vi "Main.vi"(11 "Module Admin":refnum<class "Delacor_lib_QMH_Cloneable Module Admin.lvclass">) -> ()   [LabVIEW 2024, in "PLC.lvlib"]
doc: "This template is based off of the Queued Message Handler design pattern and the Queued Message Handler project template that ships with LabVIEW.\n\nThe main difference is that the queue is private to this module and communication between modules is performed via Broadcast and Request events.\n\nRequest events are wrapped in public API methods and are handled in the Event Handling Loop (EHL) of this VI. Any module can register for Broadcast events sent by this module. The EHL generates messages based on user interface actions.\n\nThe Message Handling Loop (MHL) processes messages generated by the EHL, or by other messages. The messages are string values, so new messages can be added easily to the Message Cases case structure in the MHL. Each message cluster can also provide an optional value for Message Data, which is a variant that can be converted to whatever message-specific data is required.\n_____\nBased on DQMH Dev Tools: Project Template 7.1.0.1503."
uses:
  PLC.lvlib
  <vilib>/Delacor/Delacor QMH/Libraries/Cloneable Module Admin_class/Delacor_lib_QMH_Cloneable Module Admin.lvclass
  C:/Program Files (x86)/National Instruments/LabVIEW 2024/vi.lib/Delacor/Delacor QMH/Libraries/Module Admin_class/Delacor_lib_QMH_Module Admin.lvclass
  Module Data--cluster.ctl
  <vilib>/Delacor/Delacor QMH/Libraries/Message Queue_class/Delacor_lib_QMH_Message Queue.lvclass/Delacor_lib_QMH_Message Queue.ctl
  <vilib>/Delacor/Delacor QMH/Libraries/Cloneable Module Admin_class/Delacor_lib_QMH_Cloneable Module Admin.lvclass/Delacor_lib_QMH_Cloneable Module Admin.ctl
  Stop Argument--cluster.ctl
  <vilib>/Delacor/Delacor QMH/Libraries/Module Admin_class/Delacor_lib_QMH_Module Admin.lvclass/Delacor_lib_QMH_Module Admin.ctl
  Set IP Argument--cluster.ctl
  Connect Argument--cluster.ctl
  Connect (Reply Payload)--cluster.ctl
  <vilib>/Utility/miscctls.llb/LVPointTypeDef.ctl
  <vilib>/Delacor/Delacor QMH/Libraries/Message Queue_class/Delacor_lib_QMH_Enqueue Message (Single).vi
  <vilib>/Delacor/Delacor QMH/Libraries/Cloneable Module Admin_class/Delacor_lib_QMH_Get Module ID.vi
  <vilib>/Delacor/Delacor QMH/Libraries/Module Admin_class/Delacor_lib_QMH_Get External Launch.vi
  <vilib>/NI/Modbus Library/API/Wrapper/Create TCP Master.vi
  <vilib>/Delacor/Delacor QMH/Libraries/Message Queue_class/Delacor_lib_QMH_Message Queue.lvclass
  <vilib>/NI/Modbus Library/API/Master/Modbus Master.lvclass
  <vilib>/NI/Modbus Library/API/Wrapper/API Main.lvlib
panel:
  out "discrete inputs":bool[](array[boolean])
  out "Timeout":bool
  out "Port":i32
  out "IP":string
  out "error out":errorcluster
  out "Status":string
  in  "Simulate EHL Error":bool
  in  "Simulate MHL Error":bool
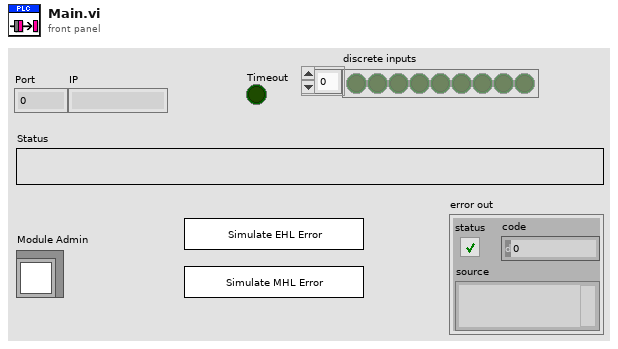
[diagram p1: front panel]
types:
  T1 = typedef "PLC.lvlib/Request Events--cluster.ctl" = cluster{"Stop Module":refnum<user-event>, "Show Panel":refnum<user-event>, "Hide Panel":refnum<user-event>, "Show Diagram":refnum<user-event>, "Get Module Execution Status":refnum<user-event>, "Set IP":refnum<user-event>, "Connect":refnum<user-event>, "Local Instance":T2}
  T2 = typedef "PLC.lvlib/Local Instance Request Events--cluster.ctl" = cluster{"Wake Up HL":refnum<user-event>}
  T3 = typedef "PLC.lvlib/Module Data--cluster.ctl" = cluster{"Status":string, "IP":string, "Port":i32}
  T4 = enum32{"invalid lock state", "Not Locked", "Locked (No Password)", "Password-protected"}
  T5 = typedef "PLC.lvlib/Stop Argument--cluster.ctl" = cluster{"Module ID":i32, "Origin":string, "Exit via Stop Module Req?":bool, "Wait for Module to stop?":bool}
  T6 = typedef "PLC.lvlib/Set IP Argument--cluster.ctl" = cluster{"Module ID":i32, "IP":string, "Port":i32}
  T7 = typedef "PLC.lvlib/Connect Argument--cluster.ctl" = cluster{"Module ID":i32, "Wait Notifier":refnum<notifier>, "wait for reply":bool}
  T8 = typedef "LVPointTypeDef.ctl" = cluster{"Horizontal":i16, "Vertical":i16}
  T9 = enum32{"Invalid", "Standard", "Closed", "Hidden", "Minimized", "Maximized"}
  T10 = typedef "PLC.lvlib/Connect (Reply Payload)--cluster.ctl" = cluster{"Module ID":i32, "Connection Status":bool, "error":errorcluster}
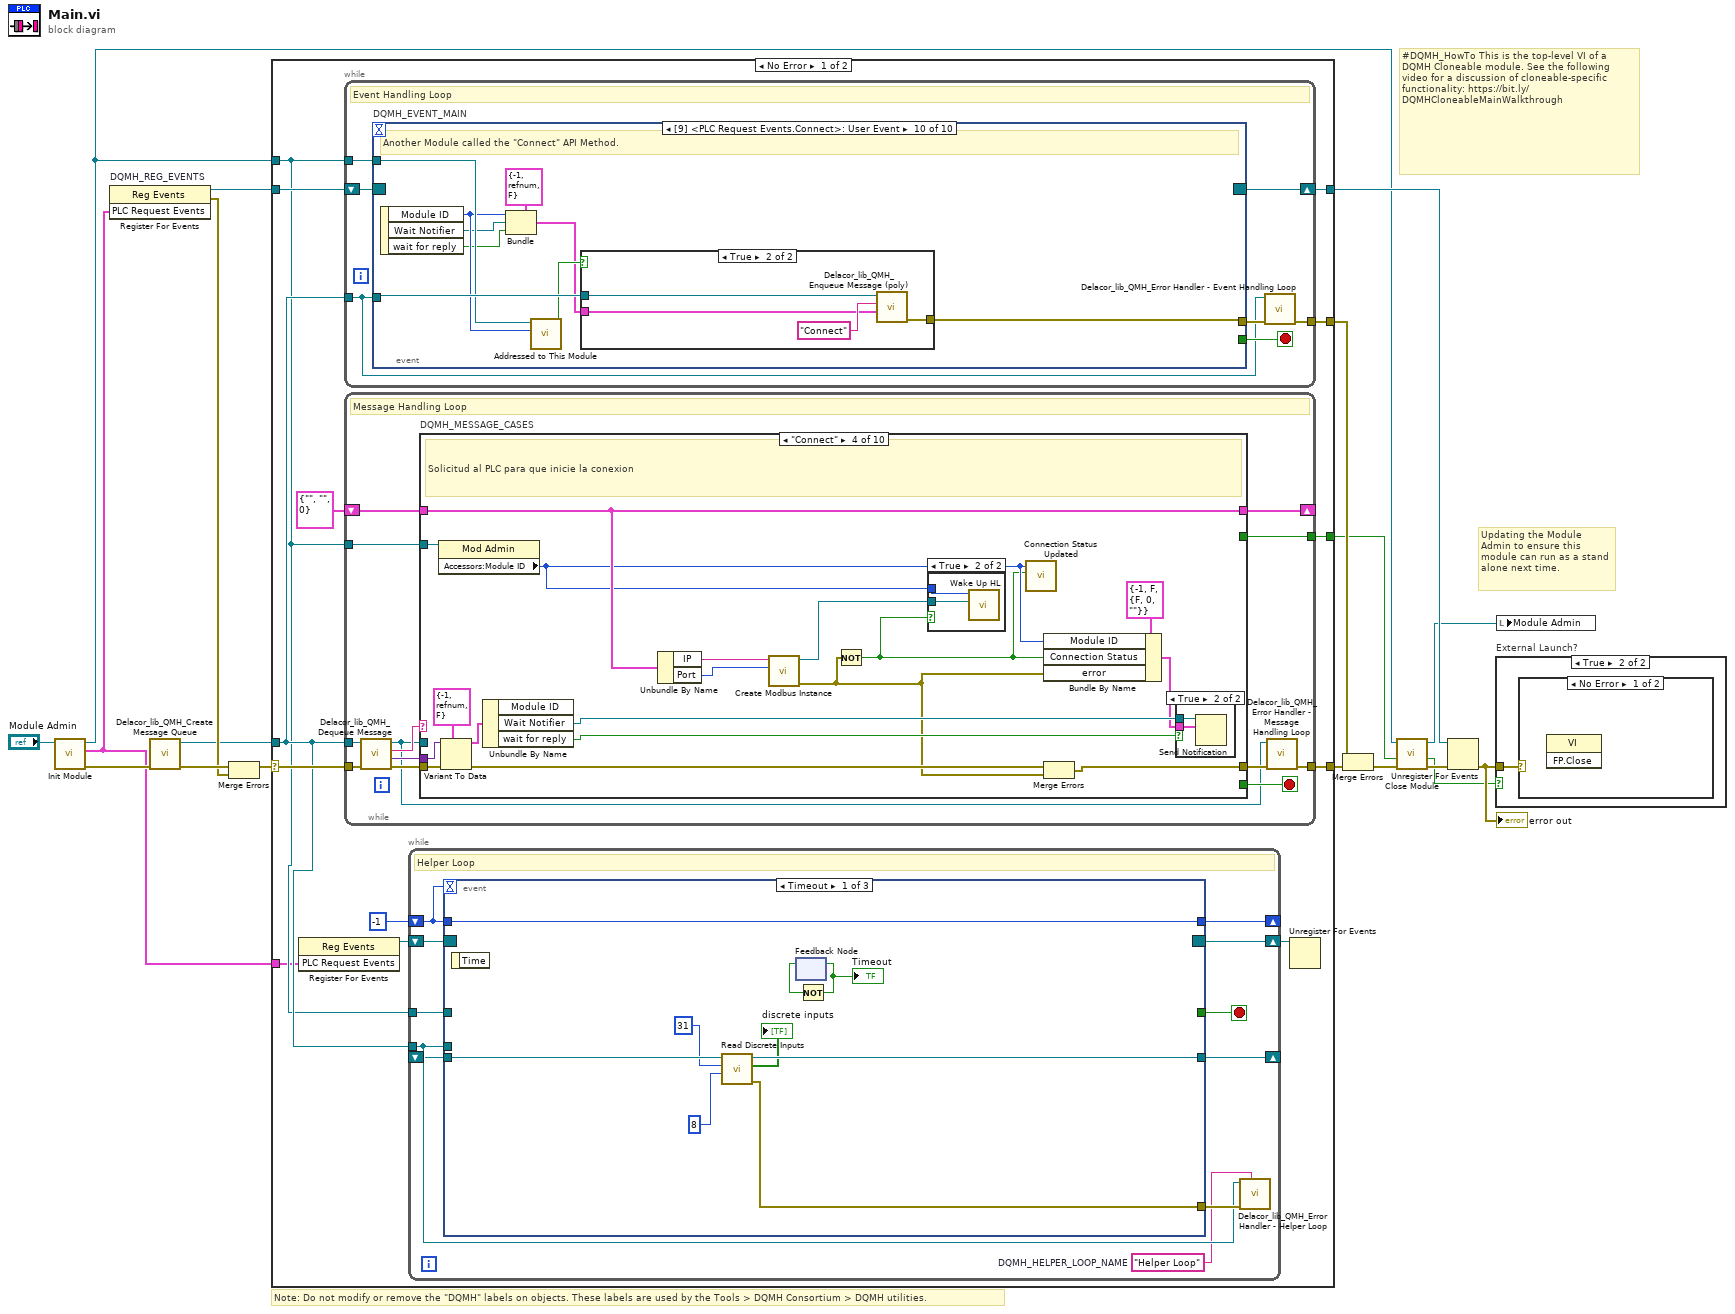
[diagram p0: block diagram]
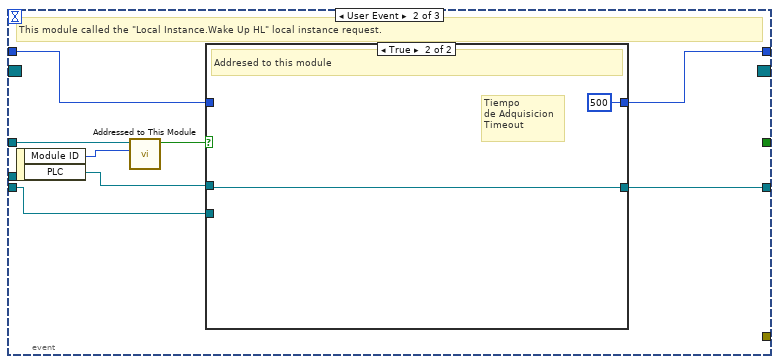
[diagram p2: hidden frame]
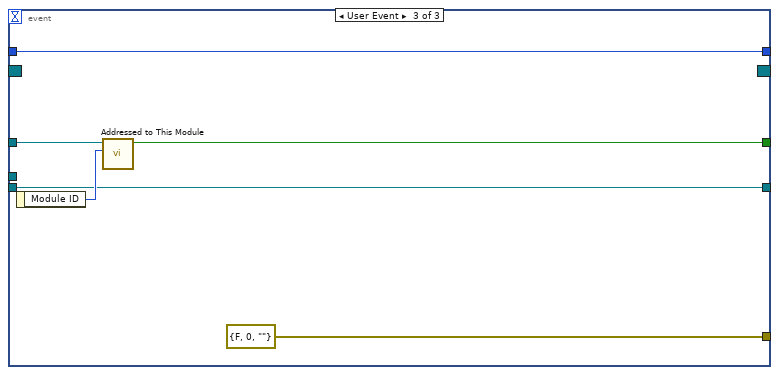
[diagram p4: hidden frame]
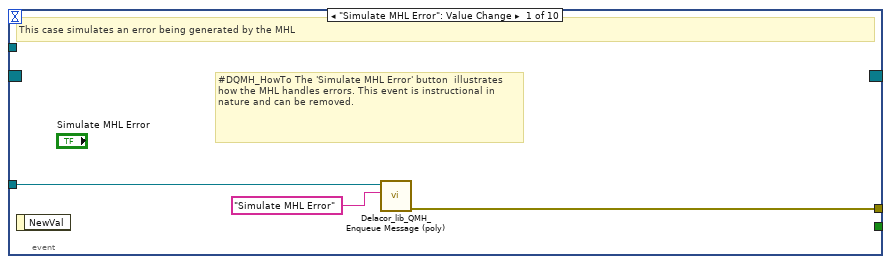
[diagram p5: hidden frame]
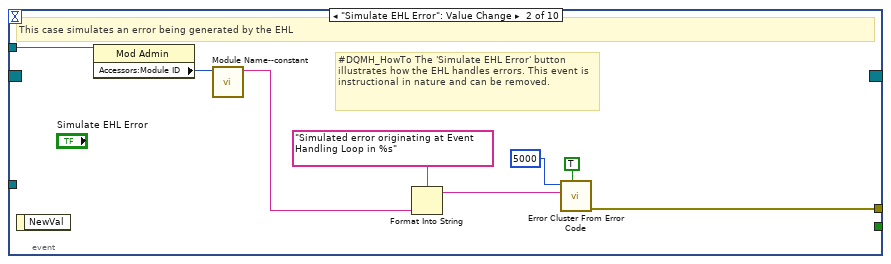
[diagram p6: hidden frame]
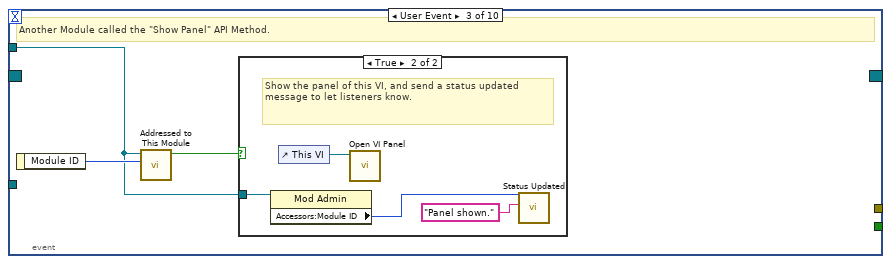
[diagram p7: hidden frame]
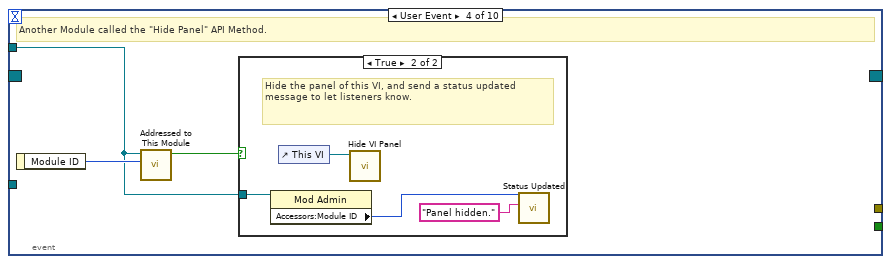
[diagram p9: hidden frame]
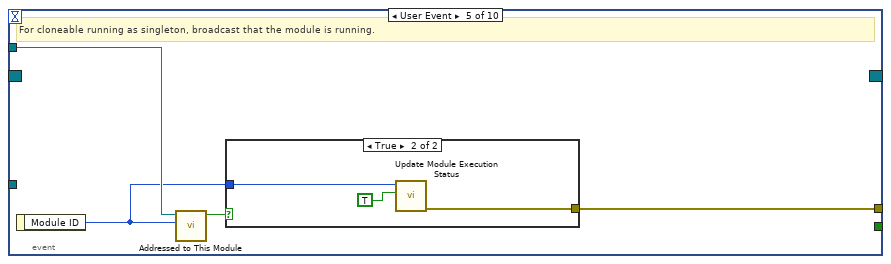
[diagram p11: hidden frame]
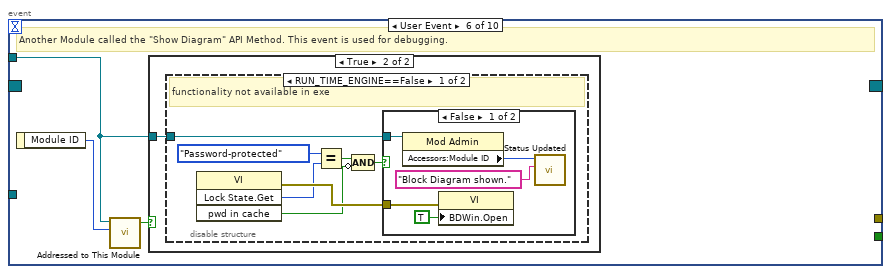
[diagram p13: hidden frame]
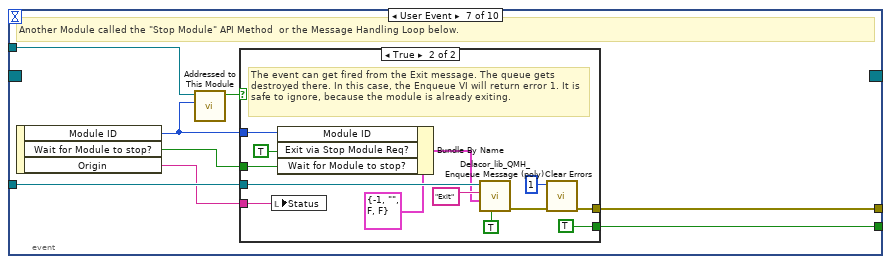
[diagram p17: hidden frame]
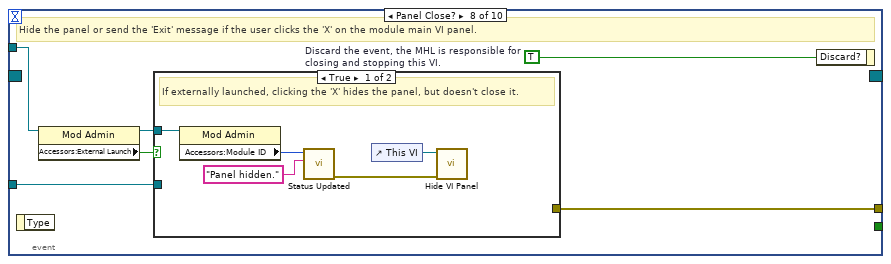
[diagram p19: hidden frame]
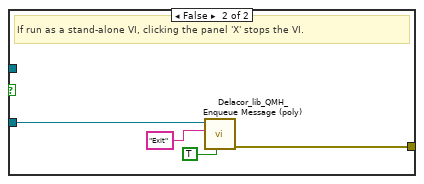
[diagram p20: hidden frame]
diagram:
  # "#DQMH_HowTo This is the top-level VI of a DQMH Cloneable module. See the following video for a discussion of cloneable-specific functionality: https://bit.ly/DQMHCloneableMainWalkthrough"
  # "Note: Do not modify or remove the \"DQMH\" labels on objects. These labels are used by the Tools > DQMH Consortium > DQMH utilities."
  # "Updating the Module Admin to ensure this module can run as a stand alone next time."
  n1 = call "Init Module.vi"("Cloneable Module Admin in"="Module Admin") -> ("error out"=w15:errorcluster, "PLC Request Events"=w1:T1, "Cloneable Module Admin out"=w5:refnum<class "Delacor_lib_QMH_Cloneable Module Admin.lvclass">)  [unwired: 8 in]
  n2 = register-events "DQMH_REG_EVENTS"(w1) -> (reference out=w8:refnum<event-registration>, error out=w10:errorcluster)  [unwired: 2 in]
  n3 = call <vilib>:"Delacor_lib_QMH_Create Message Queue.vi"("error in"=w15) -> ("error out"=w12:errorcluster, "Message Queue"=w7:refnum<class "Delacor_lib_QMH_Message Queue.lvclass">)  [unwired: 9 in]
  n4 = Merge Errors(w12, w10) -> (w11:errorcluster)
  n5 = case shown="No Error" w11 {
    selector: w11 -> [w29 w331]
    tunnel: [w31 w330] -> w16
    tunnel: [w28 w329] -> w9
    tunnel: w8 -> [w26 w329]
    tunnel: w7 -> [w25 w322]
    tunnel: [w30 _] -> w17
    tunnel: w5 -> [w24 w325]
    tunnel: [w23 _] -> w3
    tunnel: w1 -> [w22 _]
    frame No Error {
      n6 = register-events ("DQMH_HELPER_REGFOREVENTS")(w22) -> (reference out=w20:refnum<event-registration>)  [unwired: 2 in, 1 out]
      n7 = while {
        tunnel: w25 -> [w70]
        shift-right: [w73] -> w28
        shift-left: w26 -> [w74]
        tunnel: [w75] -> w30
        tunnel: w24 -> [w71]
        stop <- w72 stop-if-true
        # "Event Handling Loop"
        n8 = event "DQMH_EVENT_MAIN" shown="[9] <PLC Request Events.Connect>: User Event" {
          selector: w74 -> [_ _ _ _ _ _ _ _ _ _]
          dyn-events: [_ _ _ _ _ _ _ _ _ _] -> w73
          timeout: _ -> [_ _ _ _ _ _ _ _ _ _]
          tunnel: [_ _ _ _ _ _ w128 _ _ _] -> w72
          tunnel: w70 -> [w78 _ _ _ _ _ w131 w148 w169 w182]
          tunnel: [w79 w87 _ _ w105 _ w132 w151 w161 w174] -> w76
          tunnel: w71 -> [_ w86 w88 w95 w103 w109 w130 w149 w167 w180]
          event "Simulate MHL Error": Value Change {
            # "#DQMH_HowTo The 'Simulate MHL Error' button  illustrates how the MHL handles errors. This event is instructional in nature and can be removed."
            # "This case simulates an error being generated by the MHL"
            n9 = event-data() -> ()  [unwired: 1 in, 1 out]
            n10 = call-poly <vilib>:"Delacor_lib_QMH_Enqueue Message (poly).vi"("Message"="Simulate MHL Error", "Message Queue in"=w78) -> ("error out"=w79:errorcluster)  [unwired: 8 in, 1 out]
          }
          event "Simulate EHL Error": Value Change {
            # "#DQMH_HowTo The 'Simulate EHL Error' button  illustrates how the EHL handles errors. This event is instructional in nature and can be removed."
            # "This case simulates an error being generated by the EHL"
            n11 = event-data() -> ()  [unwired: 1 in, 1 out]
            n12 = property on="Property Node" class="Mod Admin"(reference=w86) -> ("Accessors:Module ID"=w85:i32)  [unwired: 1 in, 2 out]
            n13 = call "Module Name--constant.vi"("Module ID"=w85) -> ("Module Name"=w80:string)  [unwired: 10 in]
            n14 = Format Into String(format string="Simulated error originating at Event Handling Loop in %s", w80) -> (resulting string=w83:string)  [unwired: 2 in, 1 out]
            n15 = call <vilib>:"Error Cluster From Error Code.vi"("show call chain? (False)"=TRUE, "error message (\"\")"=w83, "error code (0)"=5000) -> ("error out"=w87:errorcluster)  [unwired: 6 in]
          }
          event User Event {
            # "Another Module called the \"Show Panel\" API Method."
            n16 = event-data() -> ("Module ID"=w89:i32)  [unwired: 1 in]
            n17 = call "Addressed to This Module.vi"("Module ID from Argument"=w89, "Module Admin"=w88) -> ("Addressed to this instance?"=w90:bool)  [unwired: 8 in, 1 out]
            n18 = case shown="True" w90 {
              tunnel: w88 -> [_ w92]
              frame False {
              }
              frame True {
                # "Show the panel of this VI, and send a status updated message to let listeners know."
                n19 = property on="Property Node" class="Mod Admin"(reference=w92) -> ("Accessors:Module ID"=w91:i32)  [unwired: 1 in, 2 out]
                n20 = control-ref of="This VI"() -> (w94:refnum<vi>)
                n21 = call "Open VI Panel.vi"("VI"=w94) -> ()  [unwired: 10 in, 1 out]
                n22 = call "Status Updated.vi"("Status"="Panel shown." ("format string"), "Module ID"=w91) -> ()  [unwired: 9 in, 1 out]
              }
            }
          }
          event User Event {
            # "Another Module called the \"Hide Panel\" API Method."
            n23 = event-data() -> ("Module ID"=w96:i32)  [unwired: 1 in]
            n24 = call "Addressed to This Module.vi"("Module ID from Argument"=w96, "Module Admin"=w95) -> ("Addressed to this instance?"=w97:bool)  [unwired: 8 in, 1 out]
            n25 = case shown="True" w97 {
              tunnel: w95 -> [_ w99]
              frame False {
              }
              frame True {
                # "Hide the panel of this VI, and send a status updated message to let listeners know."
                n26 = property on="Property Node" class="Mod Admin"(reference=w99) -> ("Accessors:Module ID"=w98:i32)  [unwired: 1 in, 2 out]
                n27 = control-ref of="This VI"() -> (w101:refnum<vi>)
                n28 = call "Hide VI Panel.vi"("VI"=w101) -> ()  [unwired: 10 in, 1 out]
                n29 = call "Status Updated.vi"("Status"="Panel hidden." ("format string"), "Module ID"=w98) -> ()  [unwired: 9 in, 1 out]
              }
            }
          }
          event User Event {
            # "For cloneable running as singleton, broadcast that the module is running."
            n30 = event-data() -> ("Module ID"=w102:i32)  [unwired: 1 in]
            n31 = call "Addressed to This Module.vi"("Module ID from Argument"=w102, "Module Admin"=w103) -> ("Addressed to this instance?"=w104:bool)  [unwired: 8 in, 1 out]
            n32 = case shown="True" w104 {
              tunnel: [_ w108] -> w105
              tunnel: w102 -> [_ w107]
              frame False {
              }
              frame True {
                n33 = call "Update Module Execution Status.vi"("Running?"=TRUE, "Module ID"=w107) -> ("error out"=w108:errorcluster)  [unwired: 9 in]
              }
            }
          }
          event User Event {
            # "Another Module called the \"Show Diagram\" API Method. This event is used for debugging."
            n34 = event-data() -> ("Module ID"=w110:i32)  [unwired: 1 in]
            n35 = call "Addressed to This Module.vi"("Module ID from Argument"=w110, "Module Admin"=w109) -> ("Addressed to this instance?"=w111:bool)  [unwired: 8 in, 1 out]
            n36 = case shown="True" w111 {
              tunnel: w109 -> [_ w112]
              frame False {
              }
              frame True {
                n37 = disable-structure shown="RUN_TIME_ENGINE==False" {
                  disable-tunnel: w112 -> [w113 _]
                  frame condition #0 (active) {
                    # "functionality not available in exe"
                    n38 = invoke on="Invoke Node" class="VI" method="Lock State.Get"() -> (error out=w119:errorcluster, "Get Lock State"=w118:T4, "pwd in cache"=w115:bool)  [unwired: 4 in, 1 out]
                    n39 = Equal?(x=T4."Password-protected", y=w118) -> (x = y?=w116:bool)
                    n40 = Compound Arithmetic op=AND(w116, invert w115) -> (w114:bool)
                    n41 = case shown="False" w114 {
                      tunnel: w119 -> [w124 _]
                      tunnel: w113 -> [w121 _]
                      frame False {
                        n42 = property on="Property Node" class="Mod Admin"(reference=w121) -> ("Accessors:Module ID"=w120:i32)  [unwired: 1 in, 2 out]
                        n43 = property on="Property Node" class="VI"(error in=w124, "BDWin.Open"=TRUE ("Block Diagram Window:Open")) -> ()  [unwired: 1 in, 2 out]
                        n44 = call "Status Updated.vi"("Status"="Block Diagram shown." ("format string"), "Module ID"=w120) -> ()  [unwired: 9 in, 1 out]
                      }
                      frame True {
                        # "Password-protected VI, and the password is not in the cache. Do not show the diagram."
                      }
                    }
                  }
                  frame condition #1 {
                  }
                }
              }
            }
          }
          event User Event {
            # "Another Module called the \"Stop Module\" API Method  or the Message Handling Loop below."
            n45 = event-data() -> ("Module ID"=w126:i32, "Wait for Module to stop?"=w127:bool, "Origin"=w125:string)  [unwired: 1 in]
            n46 = call "Addressed to This Module.vi"("Module ID from Argument"=w126, "Module Admin"=w130) -> ("Addressed to this instance?"=w129:bool)  [unwired: 8 in, 1 out]
            n47 = case shown="True" w129 {
              tunnel: [_ w144] -> w132
              tunnel: w131 -> [_ w140]
              tunnel: [_ TRUE] -> w128
              tunnel: w127 -> [_ w135]
              tunnel: w126 -> [_ w137]
              tunnel: w125 -> [_ w133]
              frame False {
              }
              frame True {
                # "The event can get fired from the Exit message. The queue gets destroyed there. In this case, the Enqueue VI will return error 1. It is safe to ignore, because the module is already exiting."
                n48 = local write "Status"(w133) -> ()
                n49 = Bundle By Name(cluster=T5 {"Module ID"=-1, "Origin"="", "Exit via Stop Module Req?"=FALSE, "Wait for Module to stop?"=FALSE} ("Stop Argument"), "Module ID"=w137, "Exit via Stop Module Req?"=TRUE, "Wait for Module to stop?"=w135) -> (w134:T5)
                n50 = call-poly <vilib>:"Delacor_lib_QMH_Enqueue Message (poly).vi"("Priority Message? (F)"=TRUE, "Message Data"=w134, "Message"="Exit", "Message Queue in"=w140) -> ("error out"=w145:errorcluster)  [unwired: 6 in, 1 out]
                n51 = call <vilib>:"Clear Errors.vi"("error in (no error)"=w145, "specific error code to clear (0: all)"=1) -> ("error out"=w144:errorcluster)  [unwired: 4 in, 1 out]
              }
            }
          }
          event Panel Close? {
            w150 = TRUE  # Discard the event, the MHL is responsible for closing and stopping this VI.
            # "Hide the panel or send the 'Exit' message if the user clicks the 'X' on the module main VI panel."
            n52 = event-data() -> ()  [unwired: 1 in, 1 out]
            n53 = property on="Property Node" class="Mod Admin"(reference=w149) -> (reference out=w146:refnum<class "Delacor_lib_QMH_Cloneable Module Admin.lvclass">, "Accessors:External Launch"=w147:bool)  [unwired: 1 in, 1 out]
            n54 = case shown="True" w147 {
              tunnel: w148 -> [_ w159]
              tunnel: [_ w160] -> w151
              tunnel: w146 -> [w154 _]
              frame True {
                # "If externally launched, clicking the 'X' hides the panel, but doesn't close it."
                n55 = property on="Property Node" class="Mod Admin"(reference=w154) -> ("Accessors:Module ID"=w153:i32)  [unwired: 1 in, 2 out]
                n56 = call "Status Updated.vi"("Status"="Panel hidden." ("format string"), "Module ID"=w153) -> ("error out"=w152:errorcluster)  [unwired: 9 in]
                n57 = control-ref of="This VI"() -> (w156:refnum<vi>)
                n58 = call "Hide VI Panel.vi"("error in"=w152, "VI"=w156) -> ()  [unwired: 9 in, 1 out]
              }
              frame False {
                # "If run as a stand-alone VI, clicking the panel 'X' stops the VI."
                n59 = call-poly <vilib>:"Delacor_lib_QMH_Enqueue Message (poly).vi"("Priority Message? (F)"=TRUE, "Message"="Exit", "Message Queue in"=w159) -> ("error out"=w160:errorcluster)  [unwired: 7 in, 1 out]
              }
            }
            n60 = event-data ("Event Filter Node")("Discard?"=w150) -> ()  [unwired: 1 in, 1 out]
          }
          event User Event {
            # "Another Module called the \"Set IP\" API Method."
            n61 = event-data() -> ("Module ID"=w164:i32, "IP"=w163:string, "Port"=w162:i32)  [unwired: 1 in]
            n62 = Bundle(cluster=T6 {"Module ID"=-1, "IP"="", "Port"=0} ("Set IP Argument"), "Module ID"=w164, "IP"=w163, "Port"=w162) -> (w165:T6)
            n63 = call "Addressed to This Module.vi"("Module ID from Argument"=w164, "Module Admin"=w167) -> ("Addressed to this instance?"=w168:bool)  [unwired: 8 in, 1 out]
            n64 = case shown="True" w168 {
              tunnel: w169 -> [_ w173]
              tunnel: w165 -> [_ w171]
              tunnel: [_ w170] -> w161
              frame False {
              }
              frame True {
                n65 = call-poly <vilib>:"Delacor_lib_QMH_Enqueue Message (poly).vi"("Message Data"=w171, "Message"="Set IP", "Message Queue in"=w173) -> ("error out"=w170:errorcluster)  [unwired: 7 in, 1 out]
              }
            }
          }
          event User Event {
            # "Another Module called the \"Connect\" API Method."
            n66 = event-data() -> ("Module ID"=w177:i32, "Wait Notifier"=w176:refnum<notifier>, "wait for reply"=w175:bool)  [unwired: 1 in]
            n67 = Bundle(cluster=T7 {"Module ID"=-1, "Wait Notifier"=refnum, "wait for reply"=FALSE} ("Connect Argument"), "Module ID"=w177, "Wait Notifier"=w176, "wait for reply"=w175) -> (w178:T7)
            n68 = call "Addressed to This Module.vi"("Module ID from Argument"=w177, "Module Admin"=w180) -> ("Addressed to this instance?"=w181:bool)  [unwired: 8 in, 1 out]
            n69 = case shown="True" w181 {
              tunnel: w182 -> [_ w186]
              tunnel: w178 -> [_ w184]
              tunnel: [_ w183] -> w174
              frame False {
              }
              frame True {
                n70 = call-poly <vilib>:"Delacor_lib_QMH_Enqueue Message (poly).vi"("Message Data"=w184, "Message"="Connect", "Message Queue in"=w186) -> ("error out"=w183:errorcluster)  [unwired: 7 in, 1 out]
              }
            }
          }
        }
        n71 = call-dynamic "Delacor_lib_QMH_Error Handler - Event Handling Loop.vi"("error in"=w76, "Message Queue in"=w70) -> ("dup error in"=w75:errorcluster)  [unwired: 8 in, 1 out]
      }
      n72 = while {
        tunnel: w25 -> [w187]
        shift-right: [w194] -> _
        shift-left: T3 {"Status"="", "IP"="", "Port"=0} ("Data Cluster") -> [w195]
        tunnel: w29 -> [w198]
        tunnel: [w196] -> w31
        tunnel: w24 -> [w189]
        tunnel: [w188] -> w23
        stop <- w193 stop-if-true
        # "Message Handling Loop"
        n73 = call-dynamic "Delacor_lib_QMH_Dequeue Message.vi"("error in"=w198, "Message Queue in"=w187) -> ("error out"=w197:errorcluster, "Message Data"=w191:variant, "Message"=w192:string, "Message Queue out"=w190:refnum<class "Delacor_lib_QMH_Message Queue.lvclass">)  [unwired: 6 in]
        n74 = case "DQMH_MESSAGE_CASES" shown="\"Connect\"" w192 {
          selector: w192 -> [_ _ _ _ _ _ _ _ _ w311]
          tunnel: w190 -> [_ _ _ _ _ _ w266 _ w303 _]
          tunnel: w197 -> [w218 w222 w236 w254 w261 w263 w275 w292 w309 w320]
          tunnel: [w216 w222 w234 w245 w260 w263 w271 w291 w304 w321] -> w199
          tunnel: w195 -> [w209 w221 w235 w243 w259 w262 w270 w289 w302 w318]
          tunnel: [w208 w221 w230 w243 w259 w262 w270 w289 w302 w318] -> w194
          tunnel: [_ _ _ _ _ _ _ _ w301 _] -> w193
          tunnel: w191 -> [_ _ w233 w252 _ _ w269 _ w299 _]
          tunnel: w189 -> [w204 _ w229 w244 _ _ w268 w287 w294 w317]
          tunnel: [_ _ _ _ _ _ _ _ w297 _] -> w188
          frame "Initialize" {
            w201 = "Initial Message" ("Initial Message")
            # "#DQMH_CodeNeeded - Initialize the appearance of the front panel."
            # "#DQMH_CodeNeeded - Initialize your state data here."
            # "Initialize - Any operation that needs to be done before the module can receive messages. Synchronize Caller Events.vi will inform Start Module.vi that the module has launched and is ready to receive messages. Module Did Init.vi will broadcast that the module initialized."
            n75 = call "Synchronize Caller Events.vi"("error in"=w218, "Module Admin"=w204) -> ("error out"=w217:errorcluster, "Module Admin out"=w203:refnum<class "Delacor_lib_QMH_Cloneable Module Admin.lvclass">)  [unwired: 8 in]
            n76 = property on="Property Node" class="Mod Admin"(reference=w203) -> ("Accessors:Module ID"=w200:i32, "Accessors:External Launch"=w205:bool)  [unwired: 1 in, 2 out]
            n77 = call "Module Name--constant.vi"("Module ID"=w200) -> ("Module Name"=w213:string)  [unwired: 10 in]
            n78 = property on="Property Node" class="VI"("Front Panel.Title"=w213) -> (reference out=w215:refnum<vi>, error out=w220:errorcluster)  [unwired: 2 in]
            n79 = Select(t=T9."Hidden" ("State"), s=w205, f=T9."Standard" ("State")) -> (s? t:f=w210:T9)
            n80 = invoke on="Invoke Node" class="VI" method="FP.Open"(reference=w215, error in=w220, "State"=w210) -> (reference out=w214:refnum<vi>, error out=w219:errorcluster)  [unwired: 2 in, 3 out]
            n81 = Bundle By Name(cluster=w209, "Status"=w201) -> (w208:T3)
            n82 = invoke on="Invoke Node" class="VI" method="FP.Center"(reference=w214, error in=w219) -> ()  [unwired: 1 in, 3 out]
            n83 = property on="Pane" class="Pane"("Origin"=T8 {"Horizontal"=0, "Vertical"=0}) -> ()  [unwired: 2 in, 2 out]
            n84 = call "Module Name--constant.vi"("Module ID"=w200) -> ("Module Name"=w206:string)  [unwired: 10 in]
            n85 = call "Module Did Init.vi"("error in"=w217, "Initialized?"=TRUE, "Origin"=w206, "Module ID"=w200) -> ("error out"=w216:errorcluster)  [unwired: 7 in]
            "Status" <- w201
          }
          frame "---Module Specific---" {
            # "Separator -- The following cases handle messages specific to this Module."
          }
          frame "Set IP" {
            # "Asignar la direccion IP para la comunicacion"
            n86 = Variant To Data(error in=w236, type=T6 {"Module ID"=-1, "IP"="", "Port"=0} ("Set IP Argument"), Variant=w233) -> (data=w231:T6, error out=w234:errorcluster)
            n87 = property class="Mod Admin"(reference=w229) -> ("Accessors:Module ID"=w224:i32)  [unwired: 1 in, 2 out]
            n88 = Unbundle By Name(w231) -> ("IP"=w228:string, "Port"=w227:i32)  [unwired: 1 out]
            "IP" <- w228
            "Port" <- w227
            n89 = Format Into String(format string="IP: %s, Port: %d", w228, w227) -> (resulting string=w226:string)  [unwired: 2 in, 1 out]
            n90 = Bundle By Name(cluster=w235, "IP"=w228, "Port"=w227) -> (w230:T3)
            n91 = call "Status Updated.vi"("Status"=w226, "Module ID"=w224) -> ()  [unwired: 9 in, 1 out]
            n92 = call "IP has been Set.vi"("IP Set"=TRUE, "Module ID"=w224) -> ()  [unwired: 9 in, 1 out]
          }
          frame "Connect" {
            # "Solicitud al PLC para que inicie la conexion"
            n93 = property class="Mod Admin"(reference=w244) -> ("Accessors:Module ID"=w238:i32)  [unwired: 1 in, 2 out]
            n94 = Variant To Data(error in=w254, type=T7 {"Module ID"=-1, "Wait Notifier"=refnum, "wait for reply"=FALSE} ("Connect Argument"), Variant=w252) -> (data=w250:T7, error out=w253:errorcluster)
            n95 = Unbundle By Name(w250) -> ("Wait Notifier"=w249:refnum<notifier>, "wait for reply"=w248:bool)  [unwired: 1 out]
            n96 = Unbundle By Name(w243) -> ("IP"=w242:string, "Port"=w241:i32)
            n97 = call-poly <vilib>:"Create Modbus Instance.vi"("port (502)"=w241, "address"=w242) -> ("error out"=w240:errorcluster, "TCP master instance"=w239:refnum<class "Modbus Master.lvclass">)  [unwired: 8 in]
            n98 = Not(x=w240) -> (.not. x?=w237:bool)
            n99 = case shown="True" w237 {
              tunnel: w239 -> [_ w256]
              tunnel: w238 -> [_ w255]
              frame False {
              }
              frame True {
                n100 = call "Wake Up HL.vi"("PLC"=w256, "Module ID"=w255) -> ()  [unwired: 9 in, 1 out]
              }
            }
            n101 = call "Connection Status Updated.vi"("Connection Status"=w237, "Module ID"=w238) -> ()  [unwired: 9 in, 1 out]
            n102 = Bundle By Name(cluster=T10 {"Module ID"=-1, "Connection Status"=FALSE, "error"={"status"=FALSE, "code"=0, "source"=""}} ("Connect (Reply Payload)"), "Module ID"=w238, "Connection Status"=w237, "error"=w240) -> (w247:T10)
            n103 = Merge Errors(w253, w240) -> (w245:errorcluster)
            n104 = case "DQMH_FIRE_NOTIFIER" shown="True" w248 {
              tunnel: w249 -> [_ w258]
              tunnel: w247 -> [_ w257]
              frame False {
              }
              frame True {
                n105 = Send Notification(notification=w257, notifier=w258) -> ()  [unwired: 1 in, 2 out]
              }
            }
          }
          frame "---Copy This Frame---" {
            # "Duplicate this frame when creating new messages.  Change this comment in the duplicated frame to describe this message."
            n106 = Merge Errors(w261) -> (w260:errorcluster)
          }
          frame "---Exit and Error Handling---" {
            # "Separator - the following cases handle errors and exit messages."
          }
          frame "Error" {
            # "#DQMH_CodeRecommended - If the module is running in standalone mode (External Launch = FALSE), this code will pop up an error dialog and call the 'Exit' message if an error occurs. Add more fine-grained error management here."
            # "Error - Check the error message data and respond accordingly. This message is sent by the \"Error Handler\" VIs at the end of each loop in this application."
            n107 = property on="Property Node" class="Mod Admin"(reference=w268) -> ("Accessors:External Launch"=w267:bool, "Accessors:Module ID"=w265:i32)  [unwired: 1 in, 2 out]
            n108 = Variant To Data(error in=w275, type=errorcluster {"status"=FALSE, "code"=0, "source"=""} ("error constant"), Variant=w269) -> (data=w264:errorcluster, error out=w273:errorcluster)
            n109 = local write "error out"(w264) -> ()
            n110 = call "Error Reported.vi"("Error"=w264, "Module ID"=w265) -> ()  [unwired: 9 in, 1 out]
            n111 = case shown="False" w267 {
              tunnel: [w280 _] -> w272
              tunnel: w266 -> [w278 _]
              tunnel: w264 -> [w279 _]
              frame False {
                n112 = disable-structure shown="Default" {
                  disable-tunnel: w279 -> [w281 _]
                  frame condition #0 (active) {
                    # "If the module is running standalone, then pop up an error dialog and call the \"Exit\" message."
                    n113 = call <vilib>:"Simple Error Handler.vi"("error in (no error)"=w281) -> ()  [unwired: 4 in, 5 out]
                  }
                  frame condition #1 {
                    # "To prevent the Simple Error Handler VI from being loaded (e.g. when deploying to a Real-Time target), add the Conditional Disable Symbol \"DQMH_Disable_SEH\" to your project and set it to TRUE."
                  }
                }
                n114 = call-poly <vilib>:"Delacor_lib_QMH_Enqueue Message (poly).vi"("Priority Message? (F)"=TRUE, "Message"="Exit", "Message Queue in"=w278) -> ("error out"=w280:errorcluster)  [unwired: 7 in, 1 out]
              }
              frame True {
                # "If the module was launched externally, calling the Error Reported broadcast VI is the only action performed by the \"Error\" message. The module's caller can then process the error appropriately."
              }
            }
            n115 = Merge Errors(w273, w272) -> (w271:errorcluster)
          }
          frame "Simulate MHL Error" {
            # "#DQMH_HowTo The 'Simulate MHL Error' button  illustrates how the MHL handles errors. This event is instructional in nature and can be removed."
            # "Simulate an error occurring at the MHL"
            n116 = property on="Property Node" class="Mod Admin"(reference=w287) -> ("Accessors:Module ID"=w288:i32)  [unwired: 1 in, 2 out]
            n117 = call "Module Name--constant.vi"("Module ID"=w288) -> ("Module Name"=w283:string)  [unwired: 10 in]
            n118 = Format Into String(format string="Simulated error originating at Message Handling Loop in %s", w283) -> (resulting string=w284:string)  [unwired: 2 in, 1 out]
            n119 = call <vilib>:"Error Cluster From Error Code.vi"("show call chain? (False)"=TRUE, "error message (\"\")"=w284, "error code (0)"=5001) -> ("error out"=w290:errorcluster)  [unwired: 6 in]
            n120 = Merge Errors(w292, w290) -> (w291:errorcluster)
          }
          frame "Exit" {
            w300 = 91  # 91: not all Exit messages will have an argument
            w301 = TRUE  # Stop the VI
            # "Release the message queue reference"
            # "#DQMH_CodeNeeded - Add any required cleanup code here."
            # "Exit - Exit the application."
            n121 = Variant To Data(error in=w309, type=T5 {"Module ID"=-1, "Origin"="", "Exit via Stop Module Req?"=FALSE, "Wait for Module to stop?"=FALSE} ("Stop Argument"), Variant=w299) -> (data=w296:T5, error out=w305:errorcluster)
            n122 = call <vilib>:"Clear Errors.vi"("error in (no error)"=w305, "specific error code to clear (0: all)"=w300) -> ("error out"=w308:errorcluster)  [unwired: 4 in, 1 out]
            n123 = property on="Property Node" class="Mod Admin"(reference=w294) -> ("Accessors:Module ID"=w293:i32)  [unwired: 1 in, 2 out]
            n124 = control-ref of="This VI"() -> (w295:refnum<vi>)
            n125 = call-dynamic "Delacor_lib_QMH_Release Message Queue.vi"("error in"=w308, "Message Queue"=w303) -> ("error out"=w307:errorcluster)  [unwired: 9 in]
            n126 = call "Handle Exit.vi"("Stop Argument"=w296, "Module Admin in"=w294, "VI reference"=w295) -> ("error out"=w306:errorcluster, "Wait for Stop?"=w297:bool)  [unwired: 7 in]
            n127 = Merge Errors(w307, w306) -> (w304:errorcluster)
            n128 = call "Error Reported.vi"("Error"=w304, "Module ID"=w293) -> ()  [unwired: 9 in, 1 out]
          }
          frame Default {
            # "'Default' case only runs if there is a message that isn't defined in any of the other cases.  Output a programming error."
            n129 = property on="Property Node" class="Mod Admin"(reference=w317) -> ("Accessors:Module ID"=w316:i32)  [unwired: 1 in, 2 out]
            n130 = call "Module Name--constant.vi"("Module ID"=w316) -> ("Module Name"=w310:string)  [unwired: 10 in]
            n131 = Format Into String(format string="The invalid message string \"%s\" was received in the Message Handling Loop for module \"%s\".", w311, w310) -> (resulting string=w313:string)  [unwired: 2 in, 1 out]
            n132 = call <vilib>:"Error Cluster From Error Code.vi"("show call chain? (False)"=TRUE, "error message (\"\")"=w313, "error code (0)"=1) -> ("error out"=w319:errorcluster)  [unwired: 6 in]
            n133 = Merge Errors(w320, w319) -> (w321:errorcluster)
          }
        }
        n134 = call-dynamic "Delacor_lib_QMH_Error Handler - Message Handling Loop.vi"("error in"=w199, "Message Queue in"=w190) -> ("dup error in"=w196:errorcluster)  [unwired: 8 in, 1 out]
      }
      n135 = while "DQMH_HELPER_LOOP" {
        shift-right: [w42] -> _
        shift-left: -1 -> [w41]
        shift-right: [w39] -> w21
        shift-left: w20 -> [w40]
        tunnel: w25 -> [w36]
        tunnel: w24 -> [w34]
        shift-right: [w33] -> _
        shift-left: _ -> [w32]
        stop <- w38 stop-if-true
        w35 = "Helper Loop"  # DQMH_HELPER_LOOP_NAME
        # "Helper Loop"
        n136 = event "DQMH_HELPER_EVENT_STRUCTURE" shown="[0] Timeout" {
          selector: w40 -> [_ _ _]
          dyn-events: [_ _ _] -> w39
          timeout: w41 -> [_ _ _]
          tunnel: w41 -> [w51 w53 w69]
          tunnel: [w51 w52 w69] -> w42
          tunnel: [_ _ w66] -> w38
          tunnel: [w43 _ errorcluster {"status"=FALSE, "code"=0, "source"=""} ("error constant")] -> w37
          tunnel: w36 -> [_ _ _]
          tunnel: w34 -> [_ w58 w67]
          tunnel: [w47 w55 w64] -> w33
          tunnel: w32 -> [w48 w54 w64]
          event Timeout {
            n137 = event-data() -> ()  [unwired: 1 in, 1 out]
            n138 = call-dynamic "Read Discrete Inputs.vi"("number of inputs"=u16 8, "starting address"=u16 31, "Modbus master in"=w48) -> ("error out"=w43:errorcluster, "discrete inputs"=→"discrete inputs":bool[], "Modbus master out"=w47:refnum<class "Modbus Master.lvclass">)  [unwired: 6 in]
            n139 = feedback #1() -> (w49:bool)  [unwired: 1 in]
            n140 = Not(x=w49) -> (.not. x?=w50:bool)
            "Timeout" <- w50
            n141 = feedback-in #1(w50) -> ()
          }
          event User Event {
            # "This module called the \"Local Instance.Wake Up HL\" local instance request."
            n142 = event-data() -> ("Module ID"=w59:i32, "PLC"=w56:refnum<class "Modbus Master.lvclass">)  [unwired: 1 in]
            n143 = call "Addressed to This Module.vi"("Module ID from Argument"=w59, "Module Admin"=w58) -> ("Addressed to this instance?"=w57:bool)  [unwired: 8 in, 1 out]
            n144 = case shown="True" w57 {
              tunnel: w56 -> [_ w63]
              tunnel: [w61 w63] -> w55
              tunnel: w54 -> [w61 _]
              tunnel: w53 -> [w60 _]
              tunnel: [w60 500] -> w52
              frame False {
              }
              frame True {
                # "Tiempo \nde Adquisicion\nTimeout"
                # "Addresed to this module"
              }
            }
          }
          event User Event {
            n145 = event-data() -> ("Module ID"=w65:i32)  [unwired: 1 in]
            n146 = call "Addressed to This Module.vi"("Module ID from Argument"=w65, "Module Admin"=w67) -> ("Addressed to this instance?"=w66:bool)  [unwired: 8 in, 1 out]
          }
        }
        n147 = call-dynamic "Delacor_lib_QMH_Error Handler - Helper Loop.vi"("Error Debug"=w35, "error in"=w37, "Message Queue in"=w36) -> ()  [unwired: 7 in, 2 out]
      }
      n148 = Unregister For Events(event registration refnum=w21) -> ()  [unwired: 1 in, 1 out]
    }
    frame Error {
      n149 = call "Synchronize Caller Events.vi"("Module Admin"=w325) -> ("Module Admin out"=w324:refnum<class "Delacor_lib_QMH_Cloneable Module Admin.lvclass">)  [unwired: 9 in, 1 out]
      n150 = property on="Property Node" class="Mod Admin"(reference=w324) -> ("Accessors:Module ID"=w323:i32)  [unwired: 1 in, 2 out]
      n151 = call-dynamic "Delacor_lib_QMH_Release Message Queue.vi"("error in"=w331, "Message Queue"=w322) -> ("error out"=w330:errorcluster)  [unwired: 9 in]
      n152 = call "Module Name--constant.vi"("Module ID"=w323) -> ("Module Name"=w328:string)  [unwired: 10 in]
      n153 = Format Into String(format string="An error occurred during initialization. %s is no longer running.", w328) -> (resulting string=w326:string)  [unwired: 2 in, 1 out]
      n154 = call "Error Reported.vi"("Additional Information"=w326, "Error"=w330, "Module ID"=w323) -> ()  [unwired: 8 in, 1 out]
    }
  }
  n155 = Merge Errors(w17, w16) -> (w18:errorcluster)
  n156 = call "Close Module.vi"("error in"=w18, "Wait for stop?"=w3, "Module Admin in"=w5) -> ("error out"=w14:errorcluster, "External Launch"=w2:bool, "Module Admin out"=w4:refnum<class "Delacor_lib_QMH_Cloneable Module Admin.lvclass">)  [unwired: 6 in]
  n157 = Unregister For Events(event registration refnum=w9, error in=w14) -> (error out=w13:errorcluster)
  "error out" <- w13
  n158 = case "External Launch?" shown="True" w2 {
    tunnel: w13 -> [_ w332]
    frame False {
    }
    frame True {
      n159 = case shown="No Error" w332 {
        frame No Error {
          n160 = invoke class="VI" method="FP.Close"() -> ()  [unwired: 3 in, 3 out]
        }
        frame Error {
          n161 = disable-structure shown="Default" {
            frame condition #0 (active) {
              n162 = invoke class="VI" method="FP.Open"("Activate"=TRUE ("Activate?")) -> ()  [unwired: 4 in, 5 out]
            }
            frame condition #1 {
              # "Don't show panel on error if running inside a built EXE."
            }
          }
        }
      }
    }
  }
  n163 = local write "Module Admin"(w4) -> ()
